vi "Preload station.vi"(0 "configuration file path":path caption="配置文件的路径", 1 "Preload station msic inf":cluster{"生产信息":refnum<vi>, "项目名称":refnum<vi>}) -> ()   [LabVIEW 2014]
uses:
  Ctl.xio/Preload station msic ctl.ctl
  SubVIS.xio/DataSocket/DataSocket_Tags.ctl
  Ctl.xio/part type.ctl
  <vilib>/Utility/file.llb/Read From Spreadsheet File (string).vi
  SubVIS.xio/DataSocket/Read PLC Vars/Read Bool Var.vi
  SubVIS.xio/DataSocket/Read PLC Vars/Read U32 Var.vi
  SubVIS.xio/DataSocket/Write PLC Vars/Write Bool Var in.vi
panel:
  in  "SQL information":string
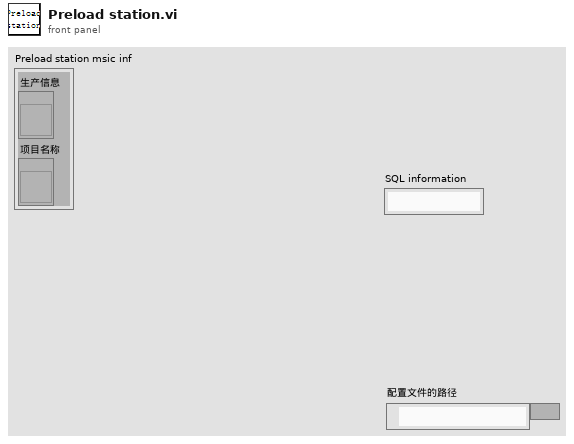
[diagram p1: front panel]
types:
  T1 = typedef "Preload station msic ctl.ctl" = cluster{"configuration file path":path, "DsOut":T2[], "Hopper car information":cluster{"Hopper car code":string, "Hopper car No":string, "plate No":string}, "pallet.produced number":i32, "SQL information":string, "Serial number":i32, "database path":path, "Preload station msic inf":cluster{"生产信息":refnum<vi>, "项目名称":refnum<vi>}, "part type":T3, "BarCode":string, "scanner resource name out":refnum<visa-resource-name>, "scanner coms":string}
  T2 = typedef "DataSocket_Tags.ctl" = cluster{"Ds ID":refnum<k13>, "Tag":string}
  T3 = typedef "part type.ctl" = cluster{"项目号":string, "物料代码":string, "零件号":string, "供应商编码":string, "产线编码":string, "客户代码":string, "颜色代码":string, "托盘上限":i32, "加热温度":string, "加热时长":string, "EOL Stations":string}
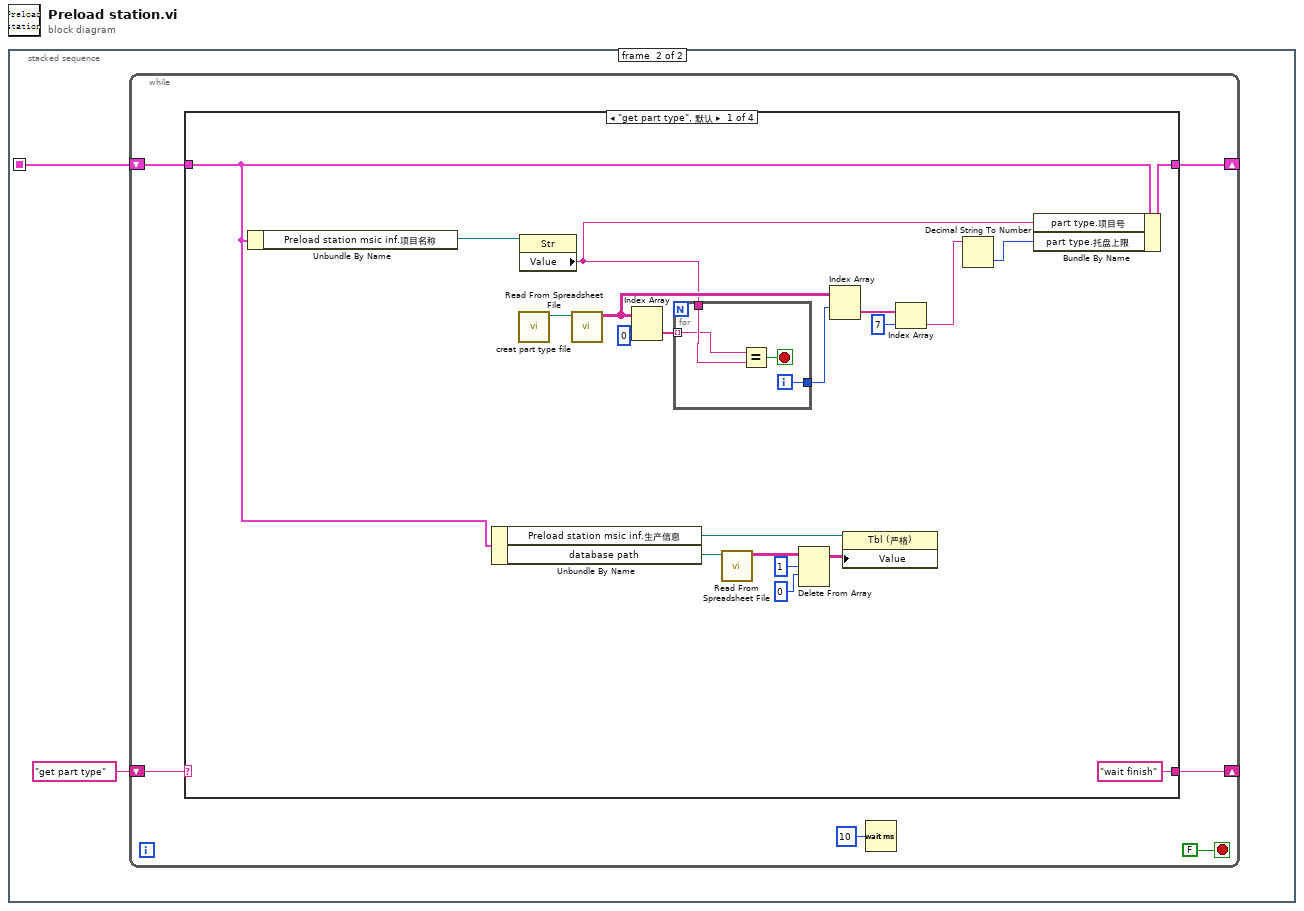
[diagram p0: block diagram]
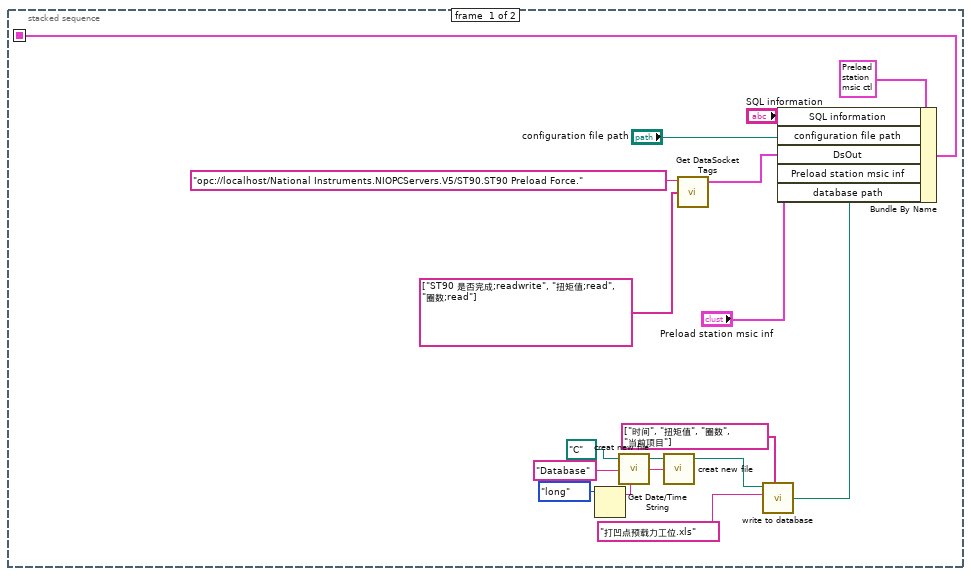
[diagram p2: hidden frame]
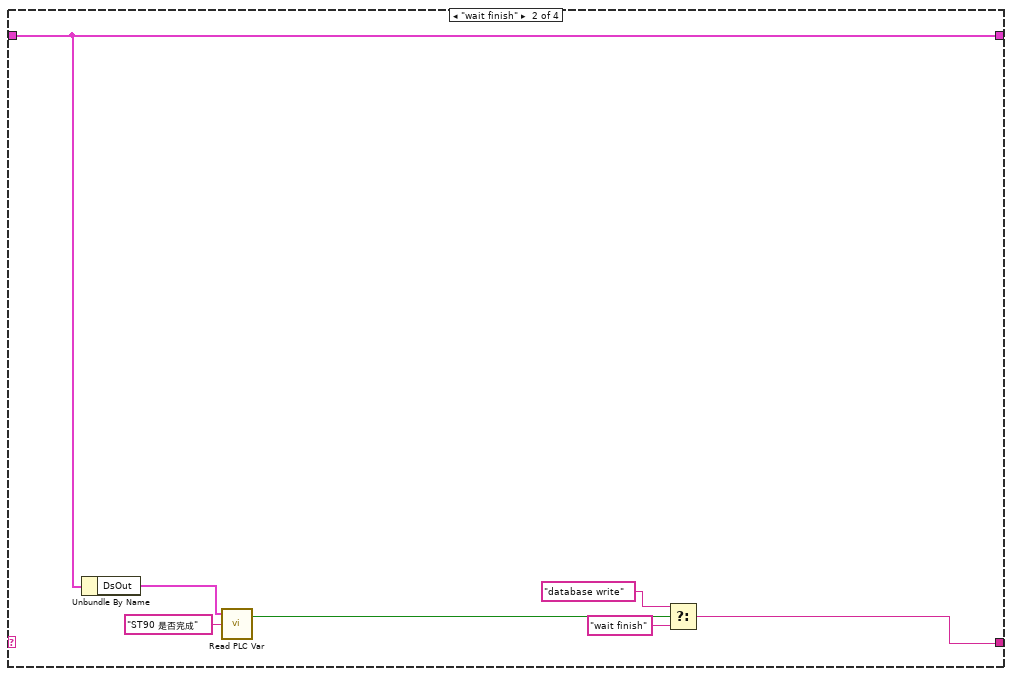
[diagram p3: hidden frame]
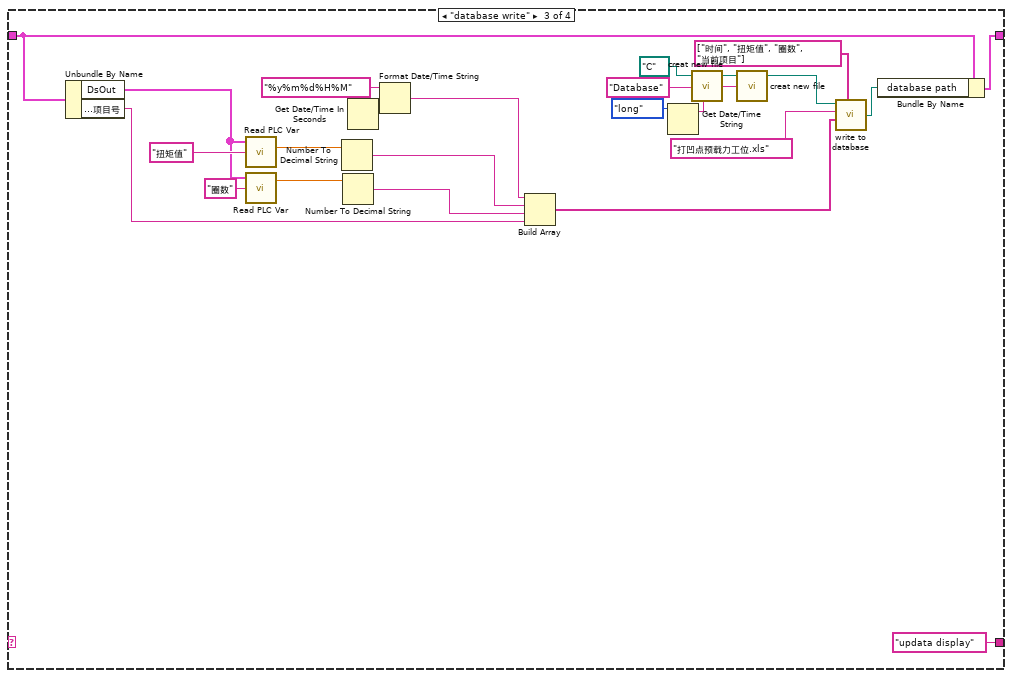
[diagram p4: hidden frame]
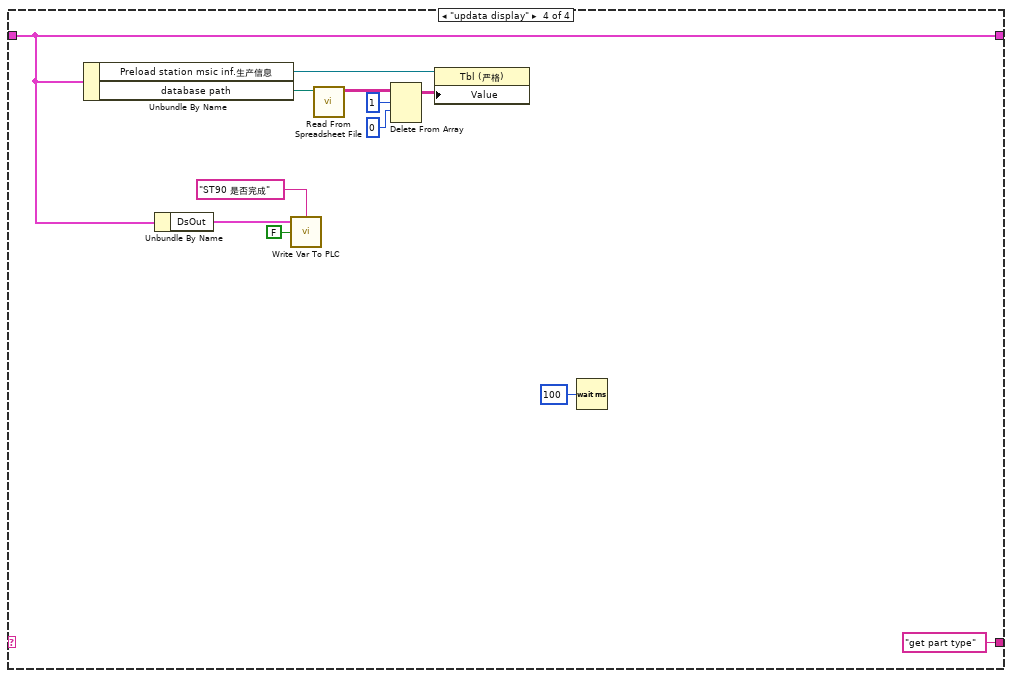
[diagram p5: hidden frame]
diagram:
  n1 = stacked-sequence {
    seq-local: [w13 _] -> [_ w19]
    frame #0 {
      n2 = Get Date/Time String(date format (0)=enum16{"short", "long", "abbreviated"}."long" ("日期格式(0)")) -> (date string=w4:string)  [unwired: 2 in, 1 out]
      n3 = call "creat new file.vi"("file name"="Database", "path"=path "C:/") -> ("created path"=w6:path)  [unwired: 1 in, 2 out]
      n4 = call "creat new file.vi"("file name"=w4, "path"=w6) -> ("created path"=w5:path)  [unwired: 1 in, 2 out]
      n5 = call "Get DataSocket Tags.vi"("All Tags"=string[] ["ST90 是否完成;readwrite", "扭矩值;read", "圈数;read"], "URL"="opc://localhost/National Instruments.NIOPCServers.V5/ST90.ST90 Preload Force.") -> ("DsOut"=w17:T2[])  [unwired: 3 in]
      n6 = call "write to database.vi"("Header"=string[] ["时间", "扭矩值", "圈数", "当前项目"], "file name"="打凹点预载力工位.xls", "path"=w5) -> ("new file path (Not A Path if cancelled)"=w1:path)  [unwired: 3 in]
      n7 = Bundle By Name(cluster=T1 {"configuration file path"=path "", "DsOut"=[], "Hopper car information"={"Hopper car code"="", "Hopper car No"="", "plate No"=""}, "pallet.produced number"=0, "SQL information"="", "Serial number"=0, "database path"=path "", "Preload station msic inf"={"生产信息"=refnum, "项目名称"=refnum}, "part type"={"项目号"="", "物料代码"="", "零件号"="", "供应商编码"="", "产线编码"="", "客户代码"="", "颜色代码"="", "托盘上限"=0, "加热温度"="", "加热时长"="", "EOL Stations"=""}, "BarCode"="", "scanner resource name out"="", "scanner coms"=""} ("PDF Welding msic ctl"), "SQL information"="SQL information", "configuration file path"="configuration file path", "DsOut"=w17, "Preload station msic inf"="Preload station msic inf", "database path"=w1) -> (w13:T1)
    }
    frame #1 {
      n8 = while {
        shift-right: [w25] -> _
        shift-left: w19 -> [w21]
        shift-right: [w24] -> _
        shift-left: "get part type" ("event") -> [w20]
        stop <- FALSE stop-if-true
        n9 = case shown="\"get part type\", 默认" w20 {
          tunnel: w21 -> [w26 w56 w71 w85]
          tunnel: [w44 w56 w75 w85] -> w25
          tunnel: ["wait finish" ("f") w51 "updata display" ("f") "get part type" ("f")] -> w24
          frame "get part type", Default {
            n10 = Unbundle By Name(w26) -> ("Preload station msic inf.项目名称"=w45:refnum<vi>)
            n11 = Unbundle By Name(w26) -> ("Preload station msic inf.生产信息"=w32:refnum<vi>, "database path"=w31:path)
            n12 = call "creat part type file.vi"() -> ("new file path (Not A Path if cancelled)"=w35:path)  [unwired: 11 in]
            n13 = property class="Str"(reference=w45) -> ("Value"=w34:string)  [unwired: 1 in, 2 out]
            n14 = call-poly <vilib>:"Read From Spreadsheet File.vi"("file path (dialog if empty)"=w35) -> ("all rows"=w40:string[][])  [unwired: 6 in, 4 out]
            n15 = Index Array(array=w40, index (col)=0 ("禁用的索引 (列)")) -> (element=w42:string[])  [unwired: 1 in]
            n16 = for {
              tunnel: w42 -> [w46] mode=indexing
              tunnel: [w48] -> w39
              tunnel: w34 -> [w47]
              i -> [w48]
              stop <- w49 stop-if-true
              n17 = Equal?(x=w46, y=w47) -> (x = y?=w49:bool)
            }
            n18 = call-poly <vilib>:"Read From Spreadsheet File.vi"("file path (dialog if empty)"=w31) -> ("all rows"=w30:string[][])  [unwired: 6 in, 4 out]
            n19 = Delete From Array(array=w30, length=1 ("长度"), index (row)=0 ("索引 (行)")) -> (array with subset deleted=w27:string[][])  [unwired: 1 in, 1 out]
            n20 = Index Array(array=w40, index (row)=w39) -> (element=w38:string[])  [unwired: 1 in]
            n21 = property class="Tbl (严格)"(reference=w32, "Value"=w27) -> ()  [unwired: 1 in, 2 out]
            n22 = Index Array(array=w38, index=7 ("索引")) -> (element=w37:string)
            n23 = Decimal String To Number(string=w37) -> (number=w36:i32)  [unwired: 2 in, 1 out]
            n24 = Bundle By Name(cluster=w26, "part type.项目号"=w34, "part type.托盘上限"=w36) -> (w44:T1)
          }
          frame "wait finish" {
            n25 = Unbundle By Name(w56) -> ("DsOut"=w55:T2[])
            n26 = call-poly "Read PLC Var.vi"("Tag IN"="ST90 是否完成", "Ds PLCTags IN"=w55) -> ("Bool Var out"=w53:bool)  [unwired: 1 in, 1 out]
            n27 = Select(t="database write" ("f"), s=w53, f="wait finish") -> (s? t:f=w51:string)
          }
          frame "database write" {
            n28 = Unbundle By Name(w71) -> ("DsOut"=w68:T2[], "part type.项目号"=w59:string)
            n29 = call-poly "Read PLC Var.vi"("Tag IN"="扭矩值", "Ds PLCTags IN"=w68) -> ("U32 Var out"=w66:dbl)  [unwired: 1 in, 1 out]
            n30 = call-poly "Read PLC Var.vi"("Tag IN"="圈数", "Ds PLCTags IN"=w68) -> ("U32 Var out"=w65:dbl)  [unwired: 1 in, 1 out]
            n31 = Number To Decimal String(number=w66) -> (decimal integer string=w64:string)  [unwired: 1 in]
            n32 = Number To Decimal String(number=w65) -> (decimal integer string=w63:string)  [unwired: 1 in]
            n33 = Get Date/Time In Seconds() -> (seconds since 1Jan1904=w62:timestamp)
            n34 = Format Date/Time String(time format string (%c)="%y%m%d%H%M" ("时间格式字符串(%c)"), seconds (now)=w62) -> (date/time string=w60:string)  [unwired: 1 in]
            n35 = Build Array(w60, w64, w63, w59) -> (w58:string[])
            n36 = Get Date/Time String(date format (0)=enum16{"short", "long", "abbreviated"}."long" ("日期格式(0)")) -> (date string=w72:string)  [unwired: 2 in, 1 out]
            n37 = call "creat new file.vi"("file name"="Database", "path"=path "C:/") -> ("created path"=w74:path)  [unwired: 1 in, 2 out]
            n38 = call "creat new file.vi"("file name"=w72, "path"=w74) -> ("created path"=w73:path)  [unwired: 1 in, 2 out]
            n39 = call "write to database.vi"("Header"=string[] ["时间", "扭矩值", "圈数", "当前项目"], "data in"=w58, "file name"="打凹点预载力工位.xls", "path"=w73) -> ("new file path (Not A Path if cancelled)"=w76:path)  [unwired: 2 in]
            n40 = Bundle By Name(cluster=w71, "database path"=w76) -> (w75:T1)
          }
          frame "updata display" {
            n41 = Unbundle By Name(w85) -> ("Preload station msic inf.生产信息"=w91:refnum<vi>, "database path"=w90:path)
            n42 = Unbundle By Name(w85) -> ("DsOut"=w84:T2[])
            n43 = call-poly "Write Var To PLC.vi"("Tag IN"="ST90 是否完成", "Bool Var in"=FALSE, "Ds PLCTags IN"=w84) -> ()  [unwired: 1 in, 2 out]
            n44 = call-poly <vilib>:"Read From Spreadsheet File.vi"("file path (dialog if empty)"=w90) -> ("all rows"=w89:string[][])  [unwired: 6 in, 4 out]
            n45 = Delete From Array(array=w89, length=1 ("长度"), index (row)=0 ("索引 (行)")) -> (array with subset deleted=w86:string[][])  [unwired: 1 in, 1 out]
            n46 = property class="Tbl (严格)"(reference=w91, "Value"=w86) -> ()  [unwired: 1 in, 2 out]
            n47 = Wait (ms)(milliseconds to wait=u32 100 ("等待时间（毫秒）")) -> ()  [unwired: 1 out]
          }
        }
        n48 = Wait (ms)(milliseconds to wait=u32 10 ("等待时间（毫秒）")) -> ()  [unwired: 1 out]
      }
    }
  }
